vi "Set Controller Configuration.vi"(8 "error in (no error)":errorcluster, 11 "Client Controller in":refnum<class "Client Controller.lvclass">) -> (0 "error out":errorcluster, 3 "Client Controller out":refnum<class "Client Controller.lvclass">)   [LabVIEW 2026, in "Client Controller.lvlib" / "Client Controller.lvclass"]
uses:
  Client Controller.lvclass
  C:/Users/E2013170/Documents/GitHub/Measurement-Utility-Reference/components/MAL-Framework/user.lib/Common Components/Controller/Controller.lvclass
  Client Config.lvclass
  MAL-Framework/user.lib/Common Components/Controller/Controller.lvclass/Controller.ctl
  Client Config.lvclass/Client Config.ctl
  Client Controller.lvclass/Client Controller.ctl
  Config/Read remote port.vi
  Config/Read IP Address of Server.vi
  MAL-Framework/user.lib/Common Components/Controller/Controller.lvclass
  Extensible-Config-Dialog/Configuration.lvclass
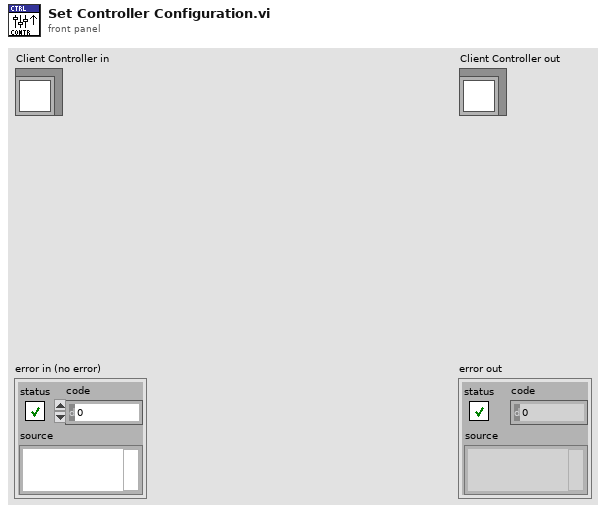
[diagram p1: front panel]
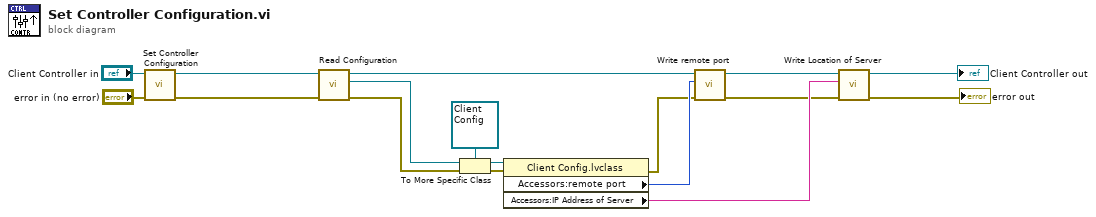
[diagram p0: block diagram]
diagram:
  n1 = call-parent "Set Controller Configuration.vi"("error in (no error)"="error in (no error)", "Controller in"="Client Controller in") -> ("error out"=w11:errorcluster, "Controller out"=w14:refnum<class "Client Controller.lvclass">)  [unwired: 8 in]
  n2 = call "Read Configuration.vi"("error in (no error)"=w11, "Controller in"=w14) -> ("error out"=w5:errorcluster, "Configuration.lvlib:Configuration.lvclass"=w10:refnum<class "Configuration.lvclass">, "Controller out"=w12:refnum<class "Client Controller.lvclass">)  [unwired: 7 in]
  n3 = To More Specific Class(target class=refnum<class "Client Config.lvclass"> refnum ("Client Controller.lvlib:Client Config.lvclass"), reference=w10, error in=w5) -> (specific class reference=w8:refnum<class "Client Config.lvclass">, error out=w4:errorcluster)
  n4 = property class="Client Config.lvclass"(reference=w8, error in=w4) -> (error out=w3:errorcluster, "Accessors:remote port"=w7:u16, "Accessors:IP Address of Server"=w6:string)  [unwired: 1 out]
  n5 = call "Write remote port.vi"("error in (no error)"=w3, "remote port"=w7, "Client Controller in"=w12) -> ("error out"=w2:errorcluster, "Client Controller out"=w15:refnum<class "Client Controller.lvclass">)  [unwired: 7 in]
  n6 = call "Write Location of Server.vi"("error in (no error)"=w2, "Location of Server"=w6, "Client Controller in"=w15) -> ("error out"=→"error out":errorcluster, "Client Controller out"=→"Client Controller out":refnum<class "Client Controller.lvclass">)  [unwired: 7 in]
